vi "Res Mirror Set State.vi"(11 "Image Acquisition Parameters":T1 {"Z Steps Size (um)" min=0.0; "Number of Z Steps" min=1; "Frames Accumulations" min=1; "Frames Per Capture" min=1; "Line Accumulations" min=1; "Image Format" items=["64 x 64"=64, "128 x 128"=128, "256 x 256"=256, "512 x 512"=512, "1024 x 1024"=1024, "2048 x 2048"=2048]}) -> (0 "Change State":bool)   [LabVIEW 2016]
uses:
  FPGA-7842R-Reference.ctl
  Type Defs/Image Acquisition Parameters.ctl
panel:
  # "Copyright (C) 2020 Edward S Allgeyer\n\nRedistribution and use in source and binary forms, with or without\nmodification, are permitted provided that the following conditions\nare met:\n\n1. Redistributions of source code must retain the above copyright\n   notice, this list of conditions and the following disclaimer.\n\n2. Redistributions in binary form must reproduce the above copyright\n   notice, this list of conditions and the following disclaimer in\n   the documentation and/or other materials provided with the\n   distribution.\n\n3. Neither the name of the copyright holder nor the names of its\n   contributors may be used to endorse or promote products derived\n   from this software without specific prior written permission.\n\nTHIS SOFTWARE IS PROVIDED BY THE COPYRIGHT HOLDERS AND CONTRIBUTORS\n\"AS IS\" AND ANY EXPRESS OR IMPLIED WARRANTIES, INCLUDING, BUT NOT\nLIMITED TO, THE IMPLIED WARRANTIES OF MERCHANTABILITY AND FITNESS\nFOR A PARTICULAR PURPOSE ARE DISCLAIMED. IN NO EVENT SHALL THE\nCOPYRIGHT HOLDER OR CONTRIBUTORS BE LIABLE FOR ANY DIRECT, INDIRECT,\nINCIDENTAL, SPECIAL, EXEMPLARY, OR CONSEQUENTIAL DAMAGES (INCLUDING,\nBUT NOT LIMITED TO, PROCUREMENT OF SUBSTITUTE GOODS OR SERVICES;\nLOSS OF USE, DATA, OR PROFITS; OR BUSINESS INTERRUPTION) HOWEVER\nCAUSED AND ON ANY THEORY OF LIABILITY, WHETHER IN CONTRACT, STRICT\nLIABILITY, OR TORT (INCLUDING NEGLIGENCE OR OTHERWISE) ARISING IN\nANY WAY OUT OF THE USE OF THIS SOFTWARE, EVEN IF ADVISED OF THE\nPOSSIBILITY OF SUCH DAMAGE."
  # "XY"
  # "Z"
  # "Length"
  # "Height"
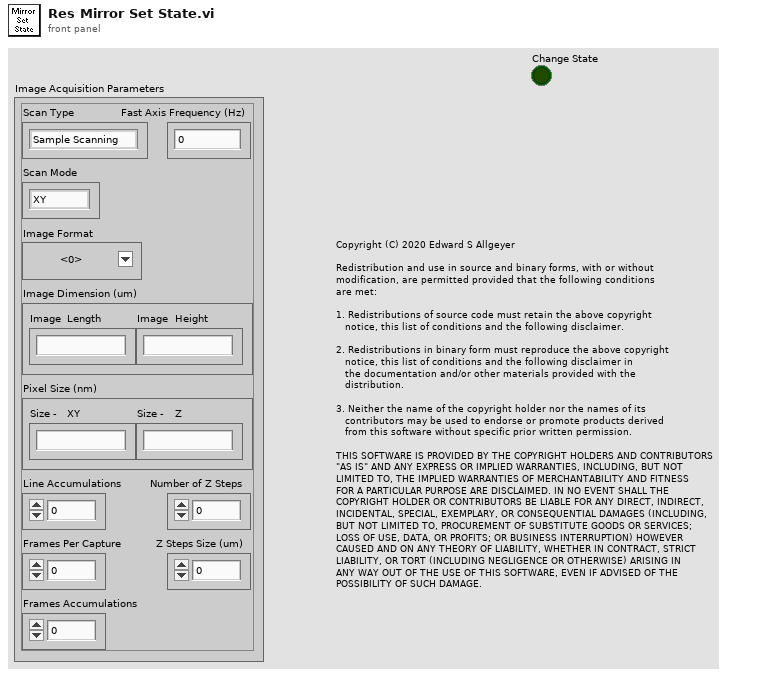
[diagram p1: front panel]
types:
  T1 = typedef "Image Acquisition Parameters.ctl" = cluster{"Scan Type":enum16{"Sample Scanning", "Beam Scanning"}, "Scan Mode":enum16{"XY", "XZ", "YZ", "XYZ"}, "Fast Axis Frequency (Hz)":dbl, "Image Format":u16, "Line Accumulations":u16, "Frames Per Capture":u16, "Frames Accumulations":u16, "Image Dimension (um)":dbl[], "Number of Z Steps":u8, "Z Steps Size (um)":dbl, "Pixel Size (nm)":dbl[]}
  T2 = typedef "Manual Controls V2.ctl" = cluster{"Galvo 1 Position (I16)":i16, "Galvo 2 Position (I16)":i16, "X Axis Voltage (I16)":i16, "Y Axis Voltage (I16)":i16, "Z Axis Voltage (I16)":i16, "Res Mirror Amp (I16)":i16, "Res Mirror Mute":bool}
  T3 = typedef "FPGA-7842R-Reference.ctl" = enum16{"Stage Control", "Laser Control", "Unused Axis I16", "Exit", "Set Res Mirror", "Set Galvo", "Default", "Close FPGA", "Stop Waveforms", "Start Waveforms", "Initialize"}
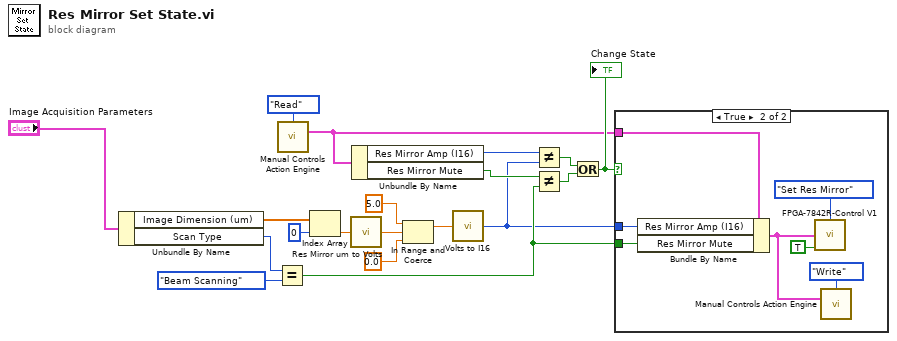
[diagram p0: block diagram]
diagram:
  n1 = Unbundle By Name("Image Acquisition Parameters") -> ("Image Dimension (um)"=w9:dbl[], "Scan Type"=w7:enum16{"Sample Scanning", "Beam Scanning"})
  n2 = Equal?(x=w7, y=enum16{"Sample Scanning", "Beam Scanning"}."Beam Scanning") -> (x = y?=w16:bool)
  n3 = call "Manual Controls Action Engine.vi"("Action"=enum16{"Read", "Write"}."Read") -> ("Manual Controls Out"=w12:T2)  [unwired: 14 in]
  n4 = Index Array(array=w9, index=0) -> (element=w5:dbl)
  n5 = call "Res Mirror um to Volts.vi"("Image Size (um)"=w5) -> ("Voltage (V)"=w4:dbl)
  n6 = Unbundle By Name(w12) -> ("Res Mirror Amp (I16)"=w13:i16, "Res Mirror Mute"=w15:bool)
  n7 = In Range and Coerce(upper limit=5.0, x=w4, lower limit=0.0) -> (coerced(x)=w3:dbl)  [unwired: 1 out]
  n8 = call "Volts to I16.vi"("Voltage (V)"=w3) -> ("I16"=w14:i16)  [unwired: 13 in, 1 out]
  n9 = Not Equal?(x=w13, y=w14) -> (x != y?=w18:bool)
  n10 = Not Equal?(x=w15, y=w16) -> (x != y?=w17:bool)
  n11 = Or(x=w18, y=w17) -> (x .or. y?=w19:bool)
  "Change State" <- w19
  n12 = case shown="True" w19 {
    tunnel: w14 -> [_ w26]
    tunnel: w16 -> [_ w21]
    tunnel: w12 -> [_ w20]
    frame False {
    }
    frame True {
      n13 = Bundle By Name(cluster=w20, "Res Mirror Amp (I16)"=w26, "Res Mirror Mute"=w21) -> (w22:T2)
      n14 = call "FPGA-7842R-Control V1.vi"("Action"=FPGA-7842R-Reference."Set Res Mirror", "Manual Controls"=w22, "Initialize"=TRUE) -> ()  [unwired: 12 in, 1 out]
      n15 = call "Manual Controls Action Engine.vi"("Action"=enum16{"Read", "Write"}."Write", "Manual Controls In"=w22) -> ()  [unwired: 13 in, 1 out]
    }
  }
